vi "XL80_v0.0.1.vi"() -> ()   [LabVIEW 2024]
uses:
  <vilib>/Utility/miscctls.llb/LVPoint32TypeDef.ctl
  Library/Class/Renishaw-XL80/Renishaw-XL80.lvclass
  Library/Class/Renishaw-XL80_EMU/Renishaw-XL80_EMU.lvclass
  <vilib>/Utility/file.llb/Write Delimited Spreadsheet (string).vi
panel:
  out "Value":dbl[](array[numeric])
  out "Numeric 2":dbl format="%.4f"
  in  "RG 2":dbl[](array[numeric]) format="%.4f"
  in  "Array":dbl[](array[numeric])
  out "Coords":T1
  in  "Table Control":string[][](table)
  in  "Read RB":bool
  out "RB":dbl[](array[numeric]) format="%.4f"
  out "RG":dbl[](array[numeric]) format="%.4f"
  in  "Reset Button":bool
  in  "Read RG":bool
  out "pStatus":i32(ring) items=["COUNT_OK"=0, "COUNT_ERROR"=1, "COUNT_TPIN_OCCURRED"=2, "COUNT_DATUMED"=4]
  in  "Connect":bool
  in  "ACM Lab ID":dbl format="%_6f"
  in  "Enter B value 2":dbl format="%_6f"
  in  "Enter Job No":dbl format="%_6f"
  in  "Listbox":i32(listbox)
  in  "?":dbl format="%_6f"
  in  "Enter mat exp coeff":dbl format="%_6f"
  in  "Export to CSV":bool
  out "Measurement":dbl format="%.4f"
  in  "Calculate_Save":bool
  out "Signal Strength":u8(slide) scale=0.0..32.0
  in  "Set Measurement Mode":i32(ring) items=["INDETERMINATE", "LINEAR_RETRO", "LINEAR_PLANE", "ANGULAR", "STRAIGHTNESS_SHORT", "STRAIGHTNESS_LONG", "VELOCITY_RETRO"]
  in  "Enter B value":dbl format="%_6f"
  out "Connected":bool
  out "Serial Number":string
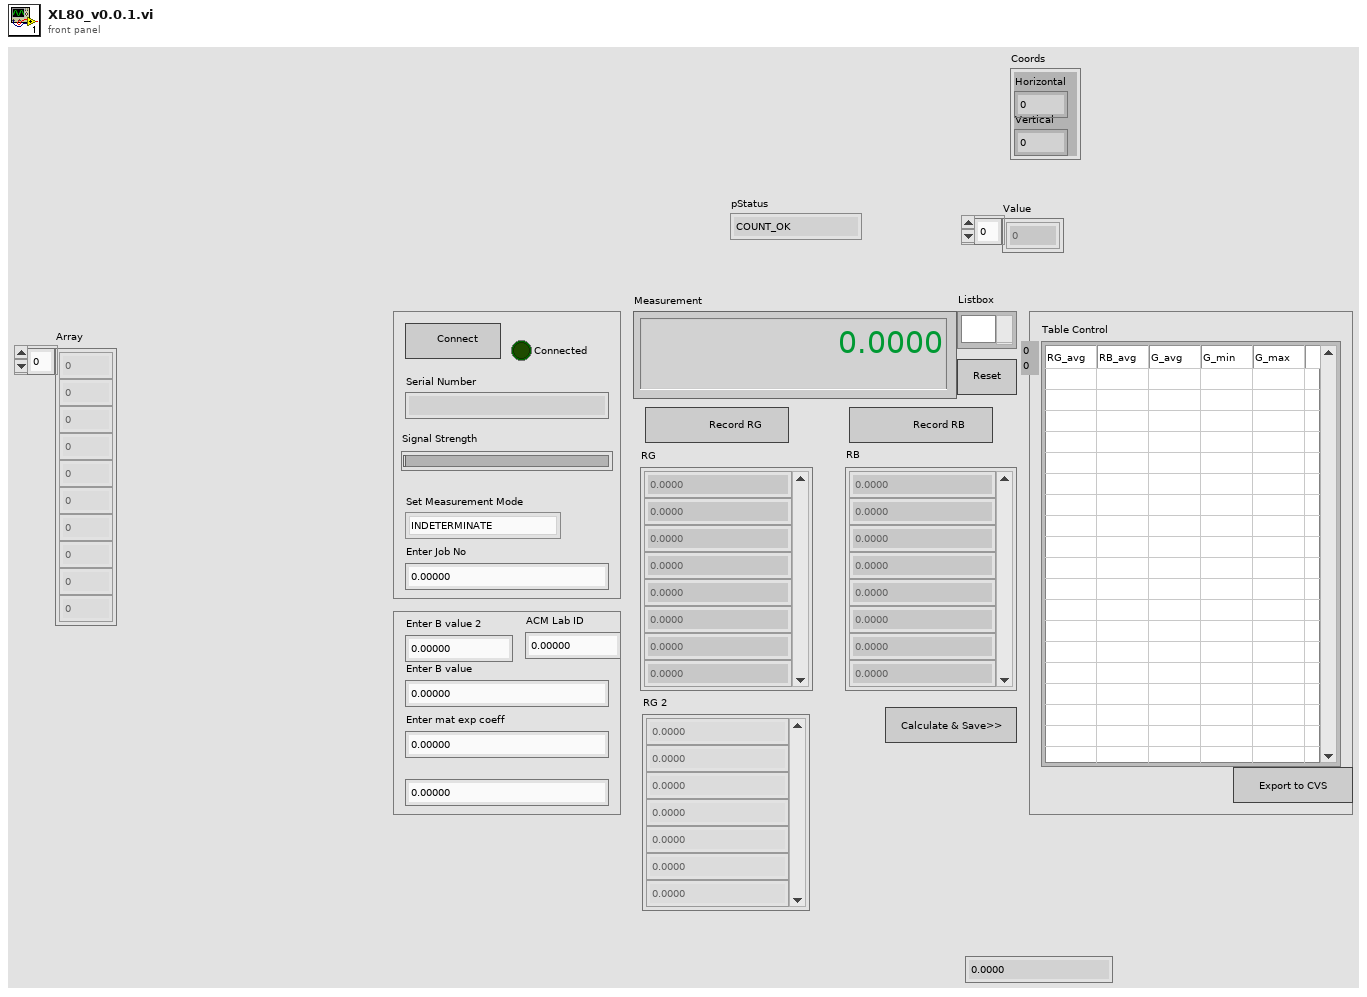
[diagram p1: front panel]
types:
  T1 = typedef "LVPoint32TypeDef.ctl" = cluster{"Horizontal":i32, "Vertical":i32}
  T2 = typedef "lveventtype.ctl" = enum32{"Null", "Timeout", "Annotation Menu Selection", "Annotation Menu Selection?", "App Instance Close", "App Instance Close?", "Autoscale Range Change", "Bookmark Info Change", "Cell Edit", "Cell Edit?", "Cursor Grab", "Cursor Grab?", "Cursor Menu Selection", "Cursor Menu Selection?", "Cursor Move", "Cursor Release", "Data Change", "Direction Change", "Display State Change", "Drag Ended", "Drag Enter", "Drag Leave", "Drag Over", "Drag Source Update", "Drag Starting", "Drag Starting?", "Drop", "Exec State Change", "Key Down", "Key Down?", "Key Repeat", "Key Repeat?", "Key Up", "Listbox Double Click", "Menu Activation?", "Menu Selection (App)", "Menu Selection? (App)", "Menu Selection (User)", "Mouse Down", "Mouse Down?", "Mouse Enter", "Mouse Leave", "Mouse Move", "Mouse Up", "Mouse Wheel", "NI Security User Change (App)", "Pane Size", "Panel Close", "Panel Close?", "Panel Resize", "Plot Attribute Change", "Scale Range Change", "Shortcut Menu Activation?", "Shortcut Menu Selection (App)", "Shortcut Menu Selection? (App)", "Shortcut Menu Selection (User)", "Tree Double Click", "Tree Drag", "Tree Drag?", "Tree Drop", "Tree Drop?", "Tree Item Close", "Tree Item Close?", "Tree Item Open", "Tree Item Open?", "User Event", "Value Change"}
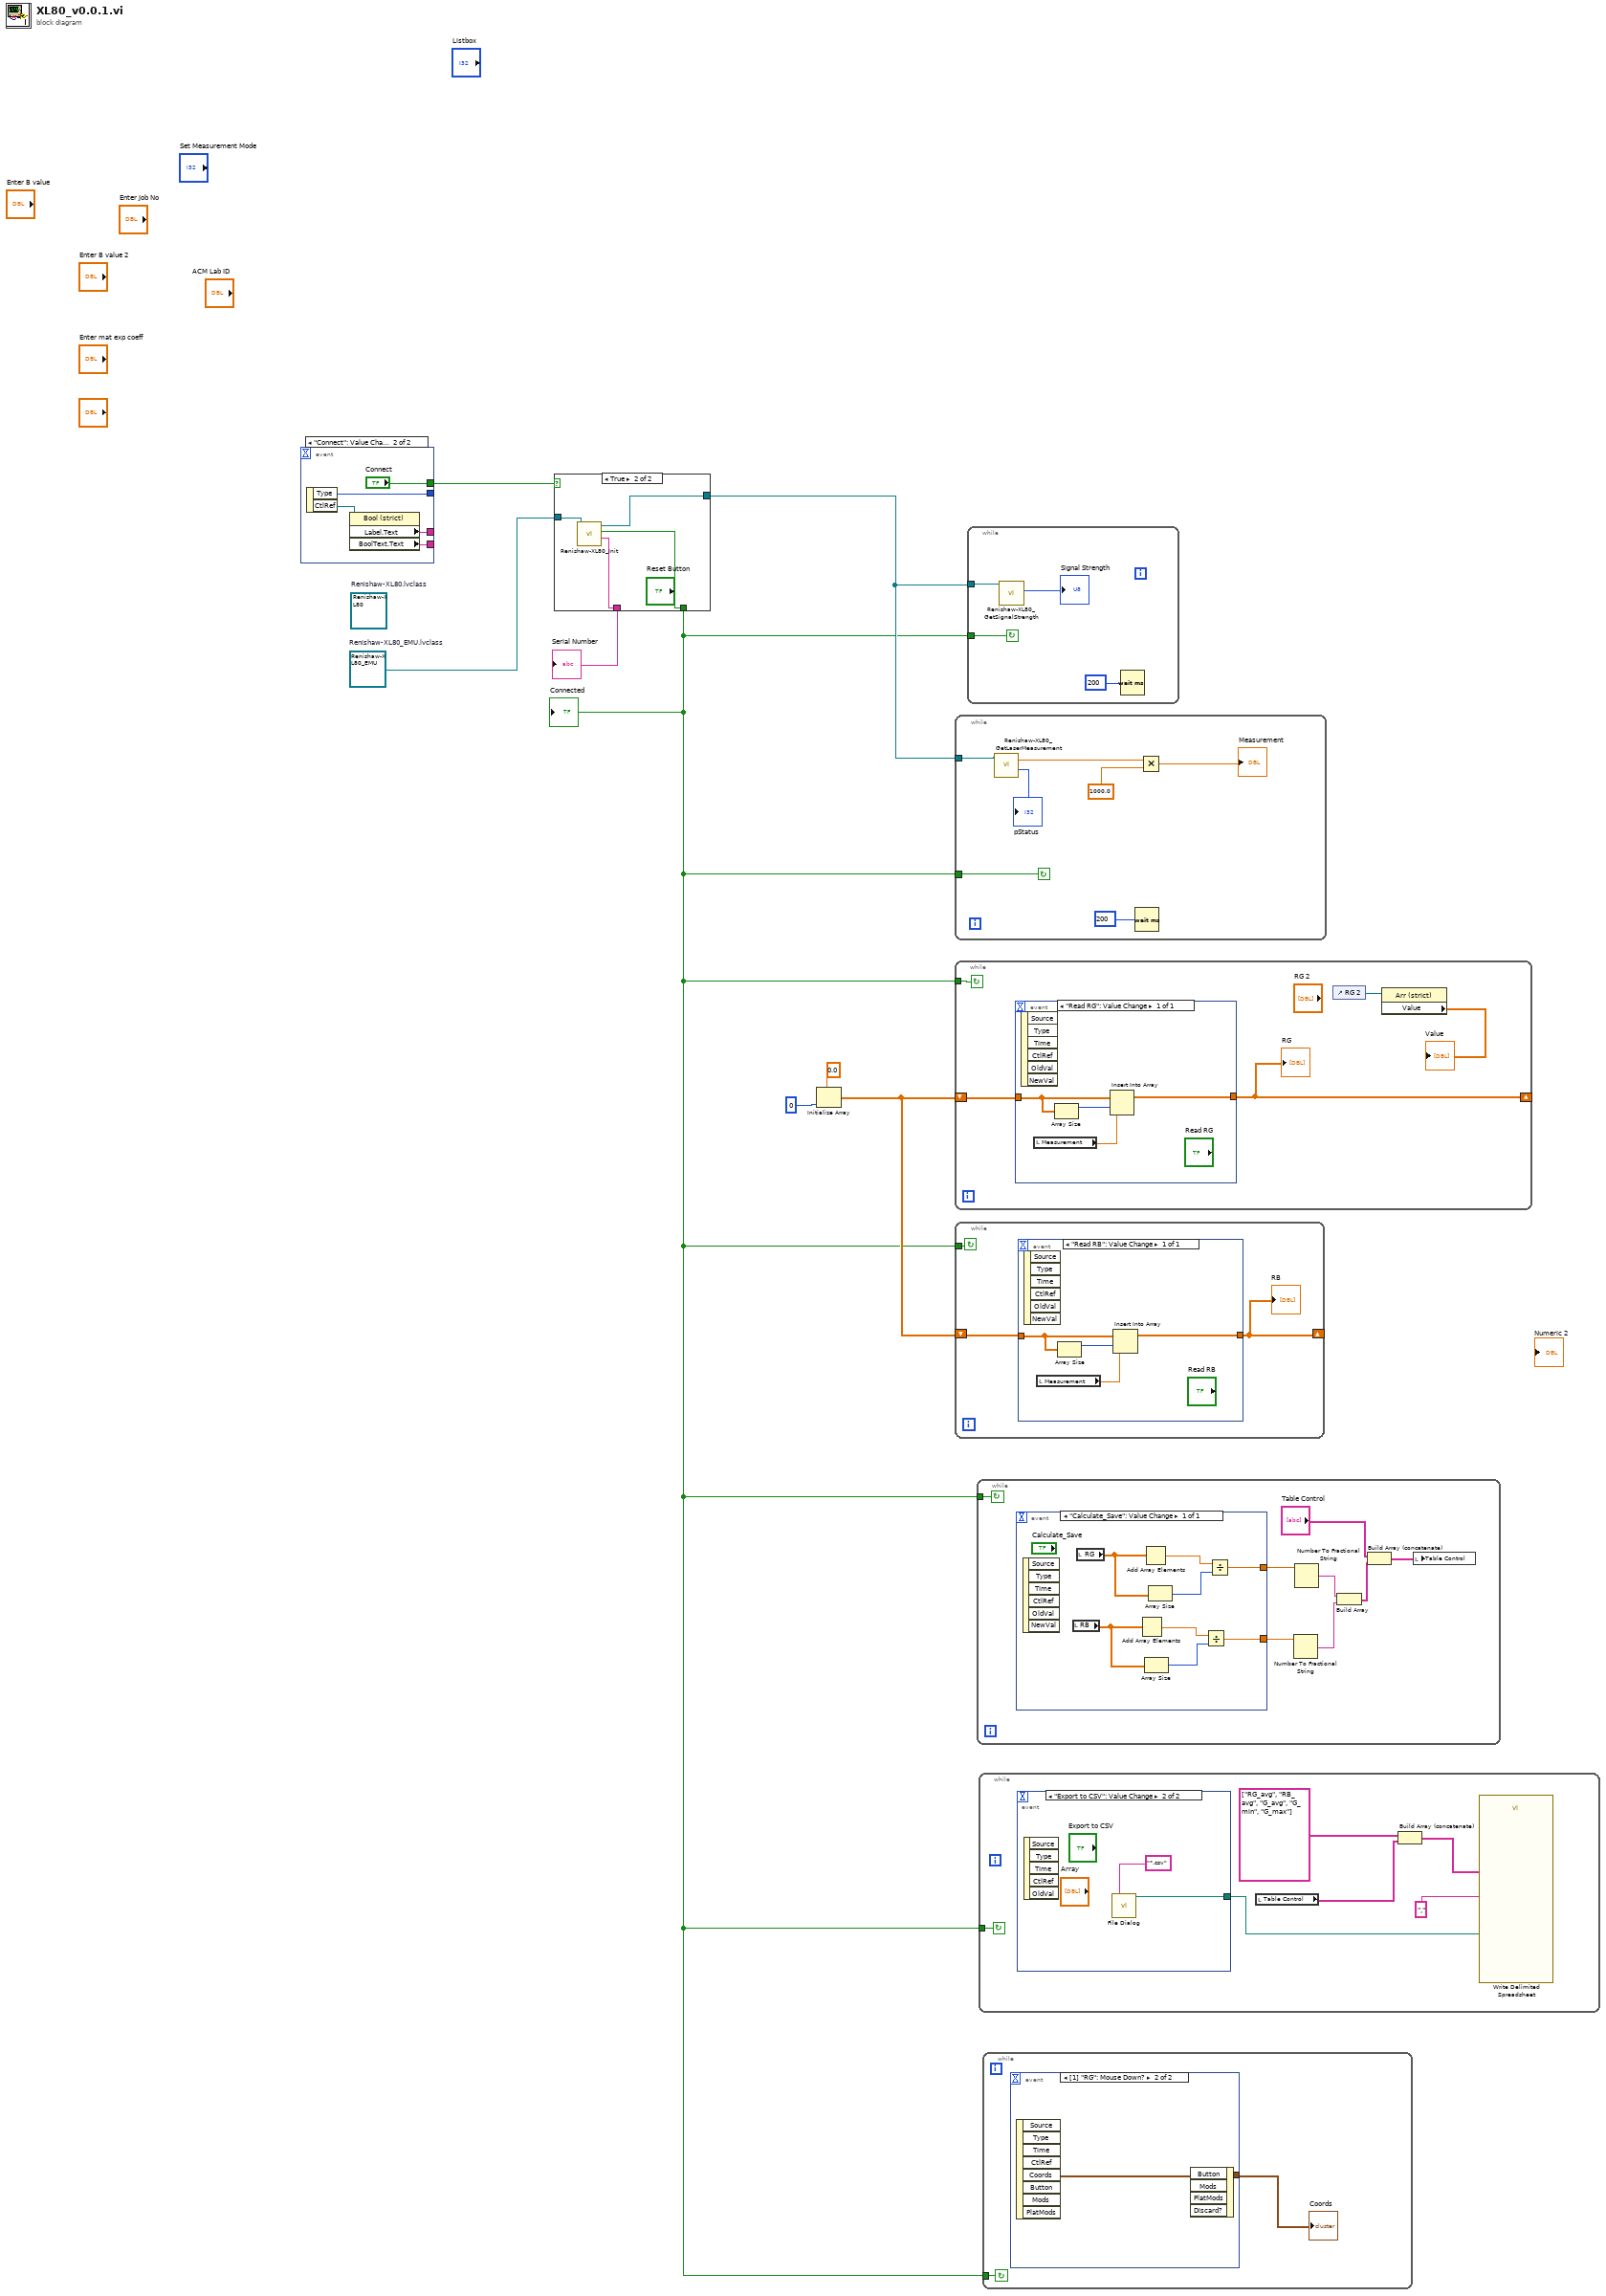
[diagram p0: block diagram]
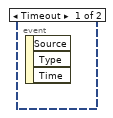
[diagram p2: hidden frame]
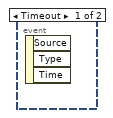
[diagram p3: hidden frame]
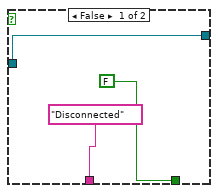
[diagram p4: hidden frame]
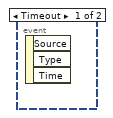
[diagram p5: hidden frame]
diagram:
  w5 = refnum<class "Renishaw-XL80_EMU.lvclass"> refnum  # Renishaw-XL80_EMU.lvclass
  (unwired) refnum<class "Renishaw-XL80.lvclass"> refnum  # Renishaw-XL80.lvclass
  n1 = event shown="[1] \"Connect\": Value Change" {
    selector: _ -> [_ _]
    dyn-events: _ -> [_ _]
    timeout: _ -> [_ _]
    tunnel: [_ w13] -> _
    tunnel: [_ w11] -> _
    tunnel: [_ w10] -> _
    tunnel: [_ "Connect"] -> w8
    event Timeout {
      n2 = event-data() -> ()  [unwired: 1 in, 3 out]
    }
    event "Connect": Value Change {
      n3 = event-data() -> ("Type"=w13:T2, "CtlRef"=w12:refnum<vi>)  [unwired: 1 in]
      n4 = property class="Bool (strict)"(reference=w12) -> ("Label.Text"=w11:string, "BoolText.Text"=w10:string)  [unwired: 1 in, 2 out]
    }
  }
  n5 = case shown="True" w8 {
    tunnel: w5 -> [w15 w20]
    tunnel: ["Disconnected" ("Serial Number") w19] -> w7
    tunnel: [w15 w18] -> w6
    tunnel: [FALSE ("Connect") w17] -> w1
    frame False {
    }
    frame True {
      n6 = call-dynamic "Renishaw-XL80_Init.vi"("Renishaw-XL80_EMU in"=w20) -> ("Serial Number"=w19:string, "Connect"=w17:bool, "Renishaw-XL80_EMU out"=w18:refnum<class "Renishaw-XL80_EMU.lvclass">)  [unwired: 7 in, 1 out]
    }
  }
  "Serial Number" <- w7
  "Connected" <- w1
  n7 = Initialize Array(0.0 ("element"), 0 ("dimension size")) -> (w2:dbl[])
  n8 = while {
    tunnel: w1 -> [w25]
    shift-right: [w21] -> _
    shift-left: w2 -> [w24]
    stop <- w25 continue-if-true
    n9 = event shown="[0] \"Read RG\": Value Change" {
      selector: _ -> [_]
      dyn-events: _ -> [_]
      timeout: _ -> [_]
      tunnel: w24 -> [w29]
      tunnel: [w26] -> w21
      event "Read RG": Value Change {
        n10 = event-data() -> ()  [unwired: 1 in, 6 out]
        n11 = local read "Measurement"() -> (w28:dbl)
        n12 = Array Size(array=w29) -> (size(s)=w27:i32)
        n13 = Insert Into Array(array=w29, index=w27, new element=w28) -> (w26:dbl[])
      }
    }
    "RG" <- w21
    n14 = control-ref of="RG 2"() -> (w23:refnum<vi>)
    n15 = property class="Arr (strict)"(reference=w23) -> ("Value"=→"Value":dbl[])  [unwired: 1 in, 2 out]
  }
  n16 = while {
    tunnel: w6 -> [w36]
    tunnel: w1 -> [w33]
    stop <- w33 continue-if-true
    n17 = call-dynamic "Renishaw-XL80_GetLaserMeasurement.vi"("Renishaw-XL80_EMU in"=w36) -> ("pStatus"=→"pStatus":i32, "GetLaserMeasurement"=w32:dbl)  [unwired: 7 in, 2 out]
    n18 = Wait (ms)(milliseconds to wait=u32 200) -> ()  [unwired: 1 out]
    n19 = Multiply(x=w32, y=1000.0) -> (x*y=→"Measurement":dbl)
  }
  n20 = while {
    tunnel: w1 -> [w39]
    shift-right: [w38] -> _
    shift-left: w2 -> [w37]
    stop <- w39 continue-if-true
    n21 = event shown="[0] \"Read RB\": Value Change" {
      selector: _ -> [_]
      dyn-events: _ -> [_]
      timeout: _ -> [_]
      tunnel: w37 -> [w43]
      tunnel: [w40] -> w38
      event "Read RB": Value Change {
        n22 = event-data() -> ()  [unwired: 1 in, 6 out]
        n23 = local read "Measurement"() -> (w42:dbl)
        n24 = Array Size(array=w43) -> (size(s)=w41:i32)
        n25 = Insert Into Array(array=w43, index=w41, new element=w42) -> (w40:dbl[])
      }
    }
    "RB" <- w38
  }
  n26 = while {
    tunnel: w6 -> [w46]
    tunnel: w1 -> [w44]
    stop <- w44 continue-if-true
    n27 = call-dynamic "Renishaw-XL80_GetSignalStrength.vi"("Renishaw-XL80_EMU in"=w46) -> ("Signal Strength"=→"Signal Strength":i16)  [unwired: 8 in, 2 out]
    n28 = Wait (ms)(milliseconds to wait=u32 200) -> ()  [unwired: 1 out]
  }
  n29 = while {
    tunnel: w1 -> [w55]
    stop <- w55 continue-if-true
    n30 = event shown="[0] \"Calculate_Save\": Value Change" {
      selector: _ -> [_]
      dyn-events: _ -> [_]
      timeout: _ -> [_]
      tunnel: [w60] -> w52
      tunnel: [w56] -> w51
      event "Calculate_Save": Value Change {
        n31 = event-data() -> ()  [unwired: 1 in, 6 out]
        n32 = local read "RB"() -> (w57:dbl[])
        n33 = local read "RG"() -> (w63:dbl[])
        n34 = Add Array Elements(numeric array=w57) -> (sum=w58:dbl)
        n35 = Add Array Elements(numeric array=w63) -> (sum=w62:dbl)
        n36 = Array Size(array=w57) -> (size(s)=w59:i32)
        n37 = Array Size(array=w63) -> (size(s)=w61:i32)
        n38 = Divide(x=w58, y=w59) -> (x/y=w56:dbl)
        n39 = Divide(x=w62, y=w61) -> (x/y=w60:dbl)
      }
    }
    n40 = Number To Fractional String(number=w51) -> (F-format string=w49:string)  [unwired: 3 in]
    n41 = Number To Fractional String(number=w52) -> (F-format string=w50:string)  [unwired: 3 in]
    n42 = Build Array(w50, w49) -> (w53:string[])
    n43 = Build Array (concatenate)("Table Control", w53) -> (w48:string[][])
    n44 = local write "Table Control"(w48) -> ()
  }
  n45 = while {
    tunnel: w1 -> [w69]
    stop <- w69 continue-if-true
    n46 = event shown="[1] \"Export to CSV\": Value Change" {
      selector: _ -> [_ _]
      dyn-events: _ -> [_ _]
      timeout: _ -> [_ _]
      tunnel: [_ w70] -> w67
      event Timeout {
        n47 = event-data() -> ()  [unwired: 1 in, 3 out]
      }
      event "Export to CSV": Value Change {
        n48 = event-data() -> ()  [unwired: 1 in, 5 out]
        n49 = call "File Dialog"("pattern (all files)"="*.csv") -> ("selected path"=w70:path)  [unwired: 11 in, 3 out]
      }
    }
    n50 = local read "Table Control"() -> (w65:string[][])
    n51 = Build Array (concatenate)(string[] ["RG_avg", "RB_avg", "G_avg", "G_min", "G_max"], w65) -> (w64:string[][])
    n52 = call-poly <vilib>:"Write Delimited Spreadsheet.vi"("file path (dialog if empty)"=w67, "2D data"=w64, "delimiter (\\t)"="," ("delimiter (\\t)")) -> ()  [unwired: 11 in, 2 out]
  }
  n53 = while {
    tunnel: w1 -> [w72]
    stop <- w72 continue-if-true
    n54 = event shown="[1] \"RG\": Mouse Down?" {
      selector: _ -> [_ _]
      dyn-events: _ -> [_ _]
      timeout: _ -> [_ _]
      tunnel: [_ w74] -> w73
      event Timeout {
        n55 = event-data() -> ()  [unwired: 1 in, 3 out]
      }
      event "RG": Mouse Down? {
        n56 = event-data() -> ("Coords"=w74:T1)  [unwired: 1 in, 7 out]
        n57 = event-data() -> ()  [unwired: 5 in, 1 out]
      }
    }
    "Coords" <- w73
  }
